vi "Inspect Fiducials.vi"(7 "Console Log in":refnum<class "Console Log.lvclass">, 8 "error in":errorcluster, 11 "Potting Procedure in":refnum<class "Potting Procedure.lvclass">) -> (0 "error out":errorcluster, 3 "Potting Procedure out":refnum<class "Potting Procedure.lvclass">, 5 "Console Log out":refnum<class "Console Log.lvclass">)   [LabVIEW 2017, in "Potting Procedure.lvclass"]
uses:
  Potting Procedure.lvclass
  Shared Components/CameraTool Class/CameraTool Class.lvclass
  Shared Components/Vec3d Class/Vec3d Class.lvclass
  <vilib>/vision/Image Controls.llb/IMAQ Image.ctl
  Shared Components/Utils/Type Definitions/Physical Image.ctl
  Type Definitions/Inspect Fiducials.ctl
  Application Utilities/Console Log/Console Log.lvclass
  Shared Components/Utils/Type Definitions/Fiducial with Source.ctl
  Shared Components/Utils/Type Definitions/Fiducial Image.ctl
  Shared Components/WorkTable Class/WorkTable Class.lvclass
  Shared Components/Gantry Class/Gantry Class.lvclass
  Shared Components/Config Manager Class/Type Definitions/Part Type.ctl
  Shared Components/FlexWorktable/FlexWorktable.lvclass
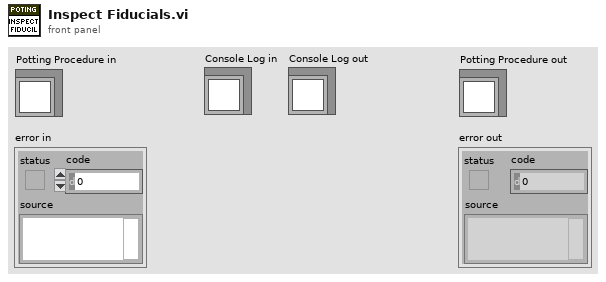
[diagram p1: front panel]
types:
  T1 = typedef "Fiducial Image.ctl" = cluster{"Fiducial Image":T2, "Selected Fiducial":T4, "fiducial name":string}
  T2 = typedef "Physical Image.ctl" = cluster{"Image Position":refnum<class "Vec3d Class.lvclass">, "Image Reference":T3, "Field of View":cluster{"x(mm)":dbl, "y(mm)":dbl}}
  T3 = typedef "IMAQ Image.ctl" = refnum<image>
  T4 = typedef "Fiducial with Source.ctl" = cluster{"Fiducial Image Coordinate":refnum<class "Vec3d Class.lvclass">, "Fiducial Source":enum16{"Pattern Recognition", "User", "Error", "Default"}}
  T5 = cluster{"Fiducials-HDI":T1[], "Fiducials-BBM":T1[], "Chuck":i32, "Slot":i32}[]
  T6 = typedef "Inspect Fiducials.ctl" = cluster{"Has Been Run?":bool, "Module-Chuck Fiducials":cluster{"Fiducials-HDI":T1[], "Fiducials-BBM":T1[], "Chuck":i32, "Slot":i32}[]}
  T7 = enum16{"Empty", "Bare HDI", "Unglued", "Stamped", "PartOnTop", "Weighted", "Unpotted", "Potted"}
  T8 = typedef "Part Type.ctl" = enum16{"BBM", "HDI", "BARE HDI", "GLUERESERVOIR", "STAMP_1", "STAMP_2", "STAMP_3", "STAMP_4", "STAMP_5", "STAMP_6", "STAMP_7", "STAMP_8", "WEIGHT_1", "WEIGHT_2", "WEIGHT_3", "WEIGHT_4", "WEIGHT_5", "WEIGHT_6", "WEIGHT_7", "WEIGHT_8", "WEIGHT_9", "WEIGHT_10", "WEIGHT_11", "WEIGHT_12", "WEIGHT_13", "WEIGHT_14", "WEIGHT_15", "WEIGHT_16", "PICKER_TOOL", "GRABER_TOOL"}
  T9 = cluster{"Fiducials-HDI":T1[], "Fiducials-BBM":T1[], "Chuck":i32, "Slot":i32}
  T10 = typedef "Worktable_Module Slot.ctl" = cluster{"Slot State":enum16{"Empty", "Bare HDI", "Unglued", "Stamped", "PartOnTop", "Weighted", "Unpotted", "Potted"}, "BBM Type":enum16{"None", "BBM", "GlassSlide"}, "HDI Type":enum16{"None", "HDI", "Polyimide"}, "Vacuum Channel":u8, "Location/Orientation BBM":T11, "Location/Orientation HDI":T11, "S/N":string}
  T11 = typedef "Position_Orientation.ctl" = cluster{"Center":refnum<class "Vec3d Class.lvclass">, "Orientation":refnum<class "Orient3d Class.lvclass">}
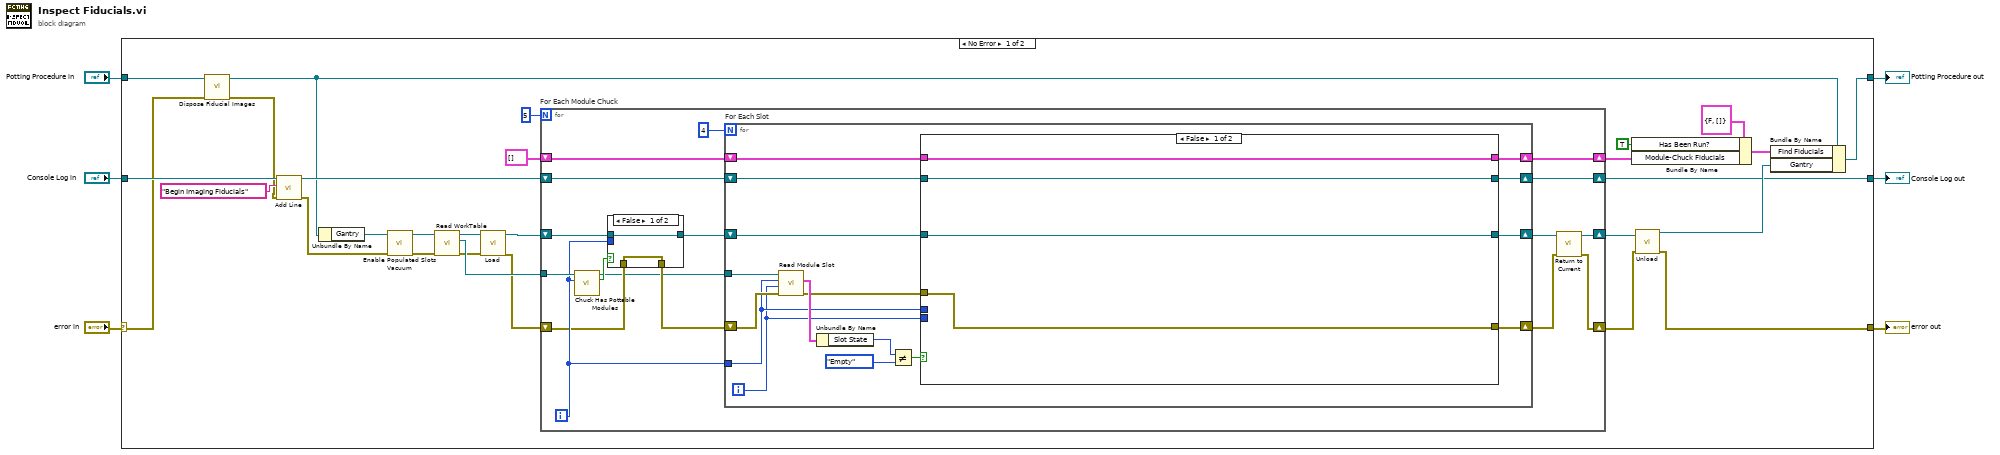
[diagram p0: block diagram]
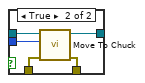
[diagram p2: hidden frame]
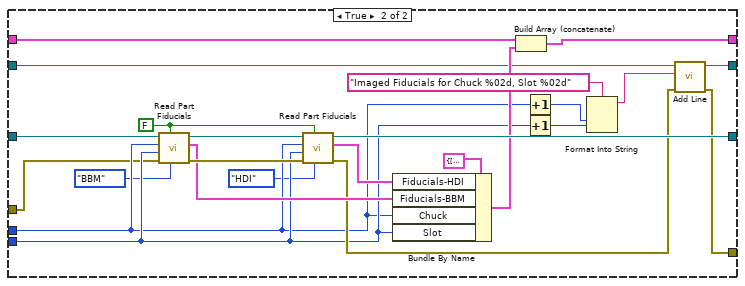
[diagram p3: hidden frame]
diagram:
  n1 = case shown="No Error" "error in" {
    selector: "error in" -> [w8 w105]
    tunnel: [w25 w105] -> w5
    tunnel: [w24 w104] -> w3
    tunnel: "Potting Procedure in" -> [w10 w104]
    tunnel: "Console Log in" -> [w18 w103]
    tunnel: [w21 w103] -> w1
    frame No Error {
      n2 = call-dynamic "Dispose Fiducial Images.vi"("error in"=w8, "Potting Procedure in"=w10) -> ("error out"=w7:errorcluster, "Potting Procedure out"=w9:refnum<class "Potting Procedure.lvclass">)  [unwired: 8 in]
      n3 = call "Add Line.vi"("error in"=w7, "String"="Begin Imaging Fiducials", "Console Log in"=w18) -> ("error out"=w12:errorcluster, "Console Log out"=w17:refnum<class "Console Log.lvclass">)  [unwired: 7 in]
      n4 = Unbundle By Name(w9) -> ("Gantry"=w14:refnum<class "Gantry Class.lvclass">)
      n5 = call-dynamic "Enable Populated Slots Vacuum.vi"("error in"=w12, "Gantry in"=w14) -> ("error out"=w11:errorcluster, "Gantry out"=w13:refnum<class "Gantry Class.lvclass">)  [unwired: 8 in]
      n6 = call-dynamic "Read WorkTable.vi"("error in"=w11, "Gantry Class in"=w13) -> ("error out"=w16:errorcluster, "Worktable"=w33:refnum<class "FlexWorktable.lvclass">, "Gantry Class out"=w34:refnum<class "Gantry Class.lvclass">)  [unwired: 7 in]
      n7 = call "Load.vi"("error in"=w16, "Gantry In"=w34) -> ("error out"=w31:errorcluster, "CameraTool out"=w30:refnum<class "CameraTool Class.lvclass">)  [unwired: 8 in]
      n8 = for "For Each Module Chuck" {
        N: 5 -> [_]
        tunnel: w33 -> [w40]
        shift-right: [w43] -> w27
        shift-left: w30 -> [w46]
        shift-right: [w41] -> w26
        shift-left: w31 -> [w37]
        shift-right: [w49] -> w19
        shift-left: T5 [] ("Module-Chuck Fiducials") -> [w50]
        shift-right: [w47] -> w21
        shift-left: w17 -> [w48]
        i -> [w39]
        n9 = call "Chuck Has Pottable Modules.vi"("Chuck"=w39, "WorkTable in"=w40) -> ("Has Pottable Modules"=w38:bool, "WorkTable out"=w35:refnum<class "WorkTable Class.lvclass">)  [unwired: 7 in, 1 out]
        n10 = case shown="False" w38 {
          tunnel: w46 -> [w53 w58]
          tunnel: [w53 w57] -> w45
          tunnel: w39 -> [_ w56]
          tunnel: w37 -> [w52 w55]
          tunnel: [w52 w54] -> w36
          frame False {
          }
          frame True {
            n11 = call-dynamic "Move To Chuck.vi"("error in"=w55, "Chuck"=w56, "Gantry in"=w58) -> ("error out"=w54:errorcluster, "Gantry out"=w57:refnum<class "CameraTool Class.lvclass">)  [unwired: 7 in]
          }
        }
        n12 = for "For Each Slot" {
          N: 4 -> [_]
          tunnel: w39 -> [w69]
          shift-right: [w66] -> w44
          shift-left: w45 -> [w70]
          shift-right: [w65] -> w42
          shift-left: w36 -> [w74]
          shift-right: [w63] -> w49
          shift-left: w50 -> [w64]
          shift-right: [w61] -> w47
          shift-left: w48 -> [w62]
          tunnel: w35 -> [w60]
          i -> [w68]
          n13 = call-dynamic "Read Module Slot.vi"("error in"=w74, "slot"=w68, "chuck"=w69, "WorkTable in"=w60) -> ("error out"=w67:errorcluster, "Module Slot"=w73:T10)  [unwired: 5 in, 1 out]
          n14 = Unbundle By Name(w73) -> ("Slot State"=w72:T7)
          n15 = Not Equal?(x=w72, y=T7."Empty") -> (x != y?=w71:bool)
          n16 = case shown="False" w71 {
            tunnel: w70 -> [w78 w80]
            tunnel: w69 -> [_ w83]
            tunnel: w68 -> [_ w85]
            tunnel: w67 -> [w77 w79]
            tunnel: [w78 w97] -> w66
            tunnel: [w77 w90] -> w65
            tunnel: w64 -> [w76 w96]
            tunnel: [w76 w94] -> w63
            tunnel: w62 -> [w75 w93]
            tunnel: [w75 w92] -> w61
            frame False {
            }
            frame True {
              w101 = FALSE ("Dispose Images?")
              n17 = call-dynamic "Read Part Fiducials.vi"("Part Type"=Part_Type."BBM", "Dispose Images?"=w101, "error in"=w79, "Slot"=w85, "Chuck"=w83, "CameraTool in"=w80) -> ("error out"=w100:errorcluster, "Fiducials"=w98:T1[], "CameraTool out"=w102:refnum<class "CameraTool Class.lvclass">)  [unwired: 3 in]
              n18 = call-dynamic "Read Part Fiducials.vi"("Part Type"=Part_Type."HDI", "Dispose Images?"=w101, "error in"=w100, "Slot"=w85, "Chuck"=w83, "CameraTool in"=w102) -> ("error out"=w91:errorcluster, "Fiducials"=w99:T1[], "CameraTool out"=w97:refnum<class "CameraTool Class.lvclass">)  [unwired: 3 in]
              n19 = Bundle By Name(cluster=T9 {"Fiducials-HDI"=[], "Fiducials-BBM"=[], "Chuck"=0, "Slot"=0} ("Module Fiducials"), "Fiducials-HDI"=w99, "Fiducials-BBM"=w98, "Chuck"=w83, "Slot"=w85) -> (w95:T9)
              n20 = Build Array (concatenate)(w96, w95) -> (w94:T5)
              n21 = Increment(x=w83) -> (x+1=w87:i32)
              n22 = Increment(x=w85) -> (x+1=w86:i32)
              n23 = Format Into String(format string="Imaged Fiducials for Chuck %02d, Slot %02d", w87, w86) -> (resulting string=w89:string)  [unwired: 2 in, 1 out]
              n24 = call "Add Line.vi"("error in"=w91, "String"=w89, "Console Log in"=w93) -> ("error out"=w90:errorcluster, "Console Log out"=w92:refnum<class "Console Log.lvclass">)  [unwired: 7 in]
            }
          }
        }
        n25 = call-dynamic "Return to Current.vi"("error in"=w42, "Gantry in"=w44) -> ("error out"=w41:errorcluster, "Gantry out"=w43:refnum<class "CameraTool Class.lvclass">)  [unwired: 8 in]
      }
      n26 = Bundle By Name(cluster=T6 {"Has Been Run?"=FALSE, "Module-Chuck Fiducials"=[]} ("Find Fiducials"), "Has Been Run?"=TRUE, "Module-Chuck Fiducials"=w19) -> (w22:T6)
      n27 = call "Unload.vi"("error in"=w26, "CameraTool in"=w27) -> ("error out"=w25:errorcluster, "Gantry out"=w23:refnum<class "Gantry Class.lvclass">)  [unwired: 8 in]
      n28 = Bundle By Name(cluster=w9, "Find Fiducials"=w22, "Gantry"=w23) -> (w24:refnum<class "Potting Procedure.lvclass">)
    }
    frame Error {
    }
  }
  "error out" <- w5
  "Potting Procedure out" <- w3
  "Console Log out" <- w1
